vi "Begin.vi"(8 "error in (no error)":errorcluster, 11 "Robot in":refnum<class "Robot.lvclass">) -> (0 "error out":errorcluster, 3 "Robot out":refnum<class "Robot.lvclass">)   [LabVIEW 2013, in "Robot.lvclass"]
uses:
  Robot.lvclass
  System/System.lvclass
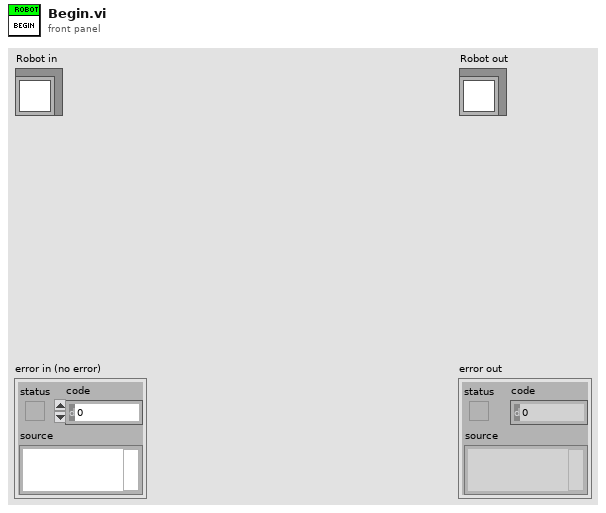
[diagram p1: front panel]
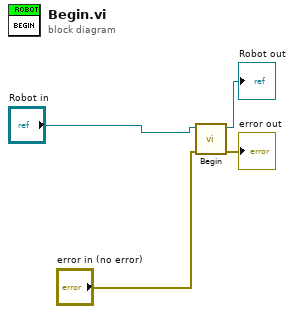
[diagram p0: block diagram]
diagram:
  n1 = call-parent "Begin.vi"("error in (no error)"="error in (no error)", "System in"="Robot in") -> ("error out"=→"error out":errorcluster, "System out"=→"Robot out":refnum<class "Robot.lvclass">)  [unwired: 8 in]
